vi "ControlesDeLaPresa.vi"() -> ()   [LabVIEW 2018]
panel:
  in  "STOP BUTTON":bool
  out "Bomba 1":dbl(knob) scale=0.0..10.0
  out "Bomba 2":dbl(knob) scale=0.0..10.0
  in  "Nivel de Agua":i32(slide) scale=0.0..100.0
  # "PRESA AVANDARO"
  # "HIGH (H)"
  # "LOW (L)"
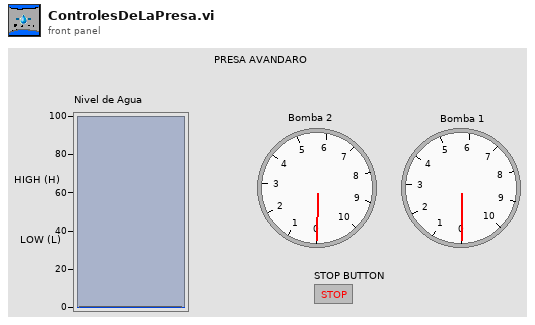
[diagram p1: front panel]
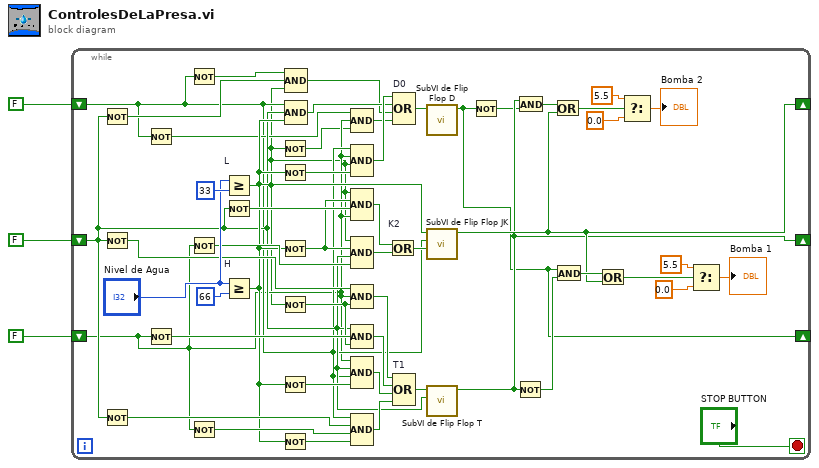
[diagram p0: block diagram]
diagram:
  n1 = while {
    shift-right: [w29] -> _
    shift-left: FALSE -> [w8]
    shift-right: [w28] -> _
    shift-left: FALSE -> [w11]
    shift-right: [w26] -> _
    shift-left: FALSE -> [w7]
    stop <- "STOP BUTTON" stop-if-true
    n2 = Not(x=w11) -> (.not. x?=w12:bool)
    n3 = Not(x=w11) -> (.not. x?=w45:bool)
    n4 = Not(x=w11) -> (.not. x?=w37:bool)
    n5 = Not(x=w8) -> (.not. x?=w9:bool)
    n6 = Not(x=w7) -> (.not. x?=w41:bool)
    n7 = Not(x=w8) -> (.not. x?=w13:bool)
    n8 = Not(x=w7) -> (.not. x?=w48:bool)
    n9 = Not(x=w7) -> (.not. x?=w36:bool)
    n10 = Greater Or Equal? "L"(x="Nivel de Agua", y=33) -> (x >= y?=w5:bool)
    n11 = Not(x=w11) -> (.not. x?=w51:bool)
    n12 = Greater Or Equal? "H"(x="Nivel de Agua", y=66) -> (x >= y?=w15:bool)
    n13 = Not(x=w5) -> (.not. x?=w6:bool)
    n14 = Not(x=w15) -> (.not. x?=w18:bool)
    n15 = Not(x=w15) -> (.not. x?=w49:bool)
    n16 = Not(x=w5) -> (.not. x?=w40:bool)
    n17 = Not(x=w15) -> (.not. x?=w39:bool)
    n18 = Not(x=w15) -> (.not. x?=w35:bool)
    n19 = Compound Arithmetic op=AND(w13, w12, w5) -> (w10:bool)
    n20 = Compound Arithmetic op=AND(w8, w11, w15) -> (w14:bool)
    n21 = Compound Arithmetic op=AND(w9, w7, w6) -> (w4:bool)
    n22 = Compound Arithmetic op=AND(w8, w7, w5, w18) -> (w17:bool)
    n23 = Compound Arithmetic op=AND(w5, w49, w51, w7) -> (w50:bool)
    n24 = Compound Arithmetic op=AND(w5, w49, w11, w48) -> (w47:bool)
    n25 = Compound Arithmetic op=AND(w45, w7, w40) -> (w44:bool)
    n26 = Compound Arithmetic op=AND(w11, w41, w40) -> (w42:bool)
    n27 = Compound Arithmetic op=AND(w7, w11, w8, w39) -> (w38:bool)
    n28 = Compound Arithmetic op=AND(w8, w37, w36, w35) -> (w34:bool)
    n29 = Or "K2"(x=w50, y=w47) -> (x .or. y?=w46:bool)
    n30 = Compound Arithmetic op=OR "D0"(w17, w14, w10, w4) -> (w16:bool)
    n31 = Compound Arithmetic op=OR "T1"(w44, w42, w38, w34) -> (w43:bool)
    n32 = call "SubVI de Flip Flop D.vi"("D0"=w16) -> ("Q0*"=w26:bool)  [unwired: 10 in]
    n33 = call "SubVI de Flip Flop JK.vi"("K"=w46, "Q2"=w8, "J"=w15) -> ("Q2*"=w29:bool)  [unwired: 8 in]
    n34 = call "SubVI de Flip Flop T.vi"("Q1"=w11, "T"=w43) -> ("Q1*"=w28:bool)  [unwired: 9 in]
    n35 = Not(x=w26) -> (.not. x?=w27:bool)
    n36 = Not(x=w28) -> (.not. x?=w30:bool)
    n37 = And(x=w28, y=w27) -> (x .and. y?=w32:bool)
    n38 = Or(x=w32, y=w29) -> (x .or. y?=w25:bool)
    n39 = And(x=w26, y=w30) -> (x .and. y?=w33:bool)
    n40 = Or(x=w33, y=w29) -> (x .or. y?=w31:bool)
    n41 = Select(t=5.5, s=w25, f=0.0) -> (s? t:f=→"Bomba 2":dbl)
    n42 = Select(t=5.5, s=w31, f=0.0) -> (s? t:f=→"Bomba 1":dbl)
  }
